vi "InsertItem.vi"(7 "Parent Tag":string, 8 "error in (no error)":errorcluster, 10 "MenuItem":refnum<class "MGI_MenuItem.lvclass">, 11 "MGI_TrayIcon in":refnum<class "MGI_TrayIcon.lvclass">) -> (0 "error out":errorcluster, 3 "MGI_TrayIcon out":refnum<class "MGI_TrayIcon.lvclass">)   [LabVIEW 2016, in "MGI_TrayIcon.lvclass"]
doc: "Authored by Derek E. Trepanier\nsupport@mooregoodideas.com\nwww.mooregoodideas.com\n\nCopyright (c) 2012, Moore Good Ideas, Inc.\n\nAll rights reserved.\n\nRedistribution and use in source and binary forms, with or without modification, are permitted provided that the following conditions are met:\n\n * Redistributions of source code must retain the above copyright notice, this list of conditions and the following disclaimer.\n * Redistributions in binary form must reproduce the above copyright notice, this list of conditions and the following disclaimer in the documentation and/or other materials provided with the distribution.\n * Neither the name of Moore Good Ideas, Inc. nor the names of its contributors may be used to endorse or promote products derived from this software without specific prior written permission.\n\nTHIS SOFTWARE IS PROVIDED BY THE COPYRIGHT HOLDERS AND CONTRIBUTORS \"AS IS\" AND ANY EXPRESS OR IMPLIED WARRANTIES, INCLUDING, BUT NOT LIMITED TO, THE IMPLIED WARRANTIES OF MERCHANTABILITY AND FITNESS FOR A PARTICULAR PURPOSE ARE DISCLAIMED. IN NO EVENT SHALL THE COPYRIGHT OWNER OR CONTRIBUTORS BE LIABLE FOR ANY DIRECT, INDIRECT, INCIDENTAL, SPECIAL, EXEMPLARY, OR CONSEQUENTIAL DAMAGES (INCLUDING, BUT NOT LIMITED TO, PROCUREMENT OF SUBSTITUTE GOODS OR SERVICES; LOSS OF USE, DATA, OR PROFITS; OR BUSINESS INTERRUPTION) HOWEVER CAUSED AND ON ANY THEORY OF LIABILITY, WHETHER IN CONTRACT, STRICT LIABILITY, OR TORT (INCLUDING NEGLIGENCE OR OTHERWISE) ARISING IN ANY WAY OUT OF THE USE OF THIS SOFTWARE, EVEN IF ADVISED OF THE POSSIBILITY OF SUCH DAMAGE."
uses:
  <userlib>/_MGI/Menu Building/MenuTypes/TrayIcon/MGI_TrayIcon.lvclass
  <userlib>/_MGI/Menu Building/MenuItem/MGI_MenuItem.lvclass
  System.Windows.Forms
  <userlib>/_MGI/Menu Building/MenuTypes/TrayIcon/MGI_TrayIcon.lvclass/MGI_TrayIcon.ctl
  <userlib>/_MGI/Menu Building/MenuItem/Read Enabled.vi
  <userlib>/_MGI/Menu Building/MenuItem/Read Checked.vi
  <userlib>/_MGI/Menu Building/MenuItem/Read Full Tag.vi
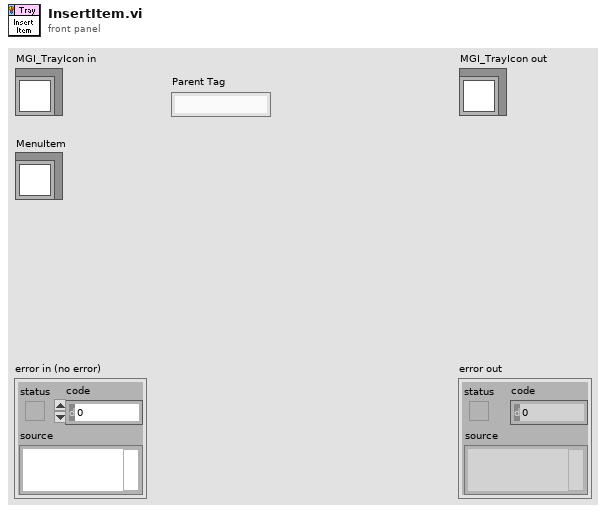
[diagram p1: front panel]
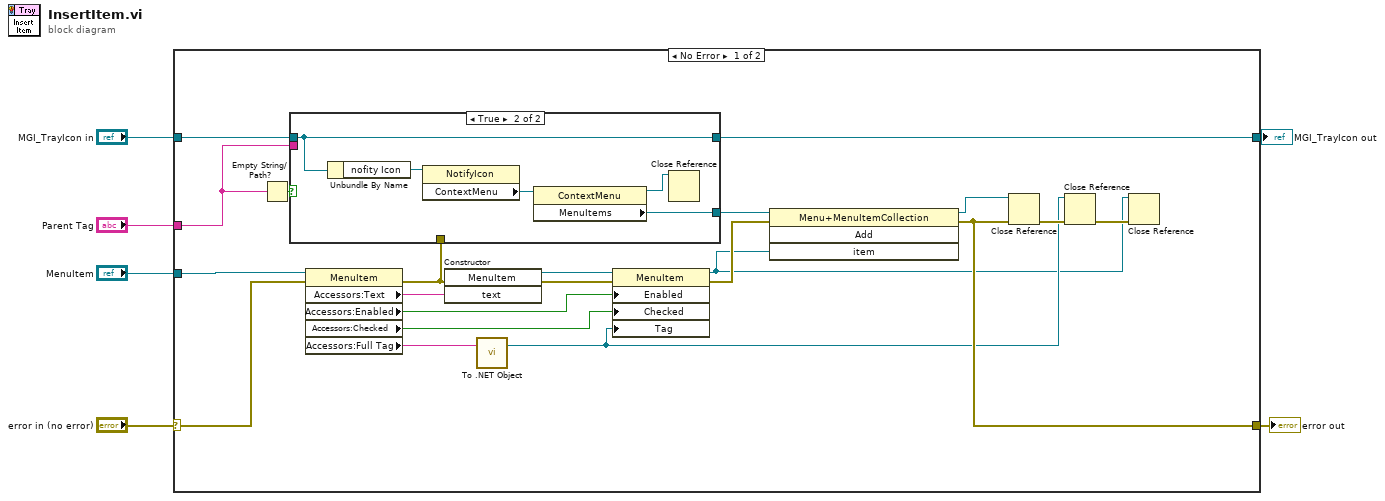
[diagram p0: block diagram]
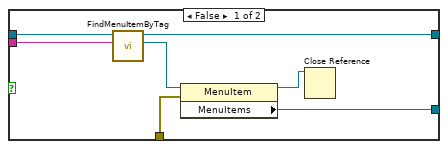
[diagram p2: hidden frame]
diagram:
  n1 = case shown="No Error" "error in (no error)" {
    selector: "error in (no error)" -> [w18 w40]
    tunnel: "MenuItem" -> [w27 _]
    tunnel: "Parent Tag" -> [w22 _]
    tunnel: "MGI_TrayIcon in" -> [w21 w41]
    tunnel: [w17 w40] -> w3
    tunnel: [w19 w41] -> w2
    frame No Error {
      n2 = Empty String/Path?(string/path=w22) -> (empty?=w12:bool)
      n3 = property class="MenuItem"(reference=w27, error in=w18) -> (error out=w24:errorcluster, "Accessors:Text"=w26:string, "Accessors:Enabled"=w8:bool, "Accessors:Checked"=w7:bool, "Accessors:Full Tag"=w9:string)  [unwired: 1 out]
      n4 = case shown="True" w12 {
        tunnel: w24 -> [w33 _]
        tunnel: w22 -> [w32 _]
        tunnel: w21 -> [w31 w37]
        tunnel: [w30 w37] -> w19
        tunnel: [w29 w36] -> w11
        frame False {
          n5 = call <userlib>:"FindMenuItemByTag.vi"("Full Tag"=w32, "NotifyIcon in"=w31) -> ("Menu Item"=w34:refnum<k24>, "NotifyIcon out"=w30:refnum<class "MGI_TrayIcon.lvclass">)  [unwired: 7 in, 1 out]
          n6 = property class="MenuItem"(reference=w34, error in=w33) -> (reference out=w28:refnum<k24>, "MenuItems"=w29:refnum<k24>)  [unwired: 1 out]
          n7 = Close Reference(reference=w28) -> ()  [unwired: 1 in, 1 out]
        }
        frame True {
          n8 = Unbundle By Name(w37) -> ("nofity Icon"=w38:refnum<k24>)
          n9 = property class="NotifyIcon"(reference=w38) -> ("ContextMenu"=w39:refnum<k24>)  [unwired: 1 in, 2 out]
          n10 = property class="ContextMenu"(reference=w39) -> (reference out=w35:refnum<k24>, "MenuItems"=w36:refnum<k24>)  [unwired: 1 in, 1 out]
          n11 = Close Reference(reference=w35) -> ()  [unwired: 1 in, 1 out]
        }
      }
      n12 = constructor class="MenuItem"(error in=w24, "text"=w26) -> (reference out=w25:refnum<k24>, error out=w23:errorcluster)  [unwired: 2 in, 2 out]
      n13 = call <vilib>:"To .NET Object.vi"("anything"=w9) -> (".NET object"=w15:refnum<k24>)  [unwired: 1 in, 1 out]
      n14 = property class="MenuItem"(reference=w25, error in=w23, "Enabled"=w8, "Checked"=w7, "Tag"=w15) -> (reference out=w13:refnum<k24>, error out=w20:errorcluster)
      n15 = invoke class="Menu+MenuItemCollection" method="Add"(reference=w11, error in=w20, "item"=w13) -> (reference out=w10:refnum<k24>, error out=w17:errorcluster)  [unwired: 1 in, 2 out]
      n16 = Close Reference(reference=w10, error in (no error)=w17) -> (error out=w16:errorcluster)
      n17 = Close Reference(reference=w15, error in (no error)=w16) -> (error out=w14:errorcluster)
      n18 = Close Reference(reference=w13, error in (no error)=w14) -> ()  [unwired: 1 out]
    }
    frame Error {
    }
  }
  "error out" <- w3
  "MGI_TrayIcon out" <- w2
